vi "Group Channels By VS and MB Type.vi"(7 "Channel Type":T1, 8 "error in (no error)":errorcluster, 11 "Item Ref in":T2 format="%.0x") -> (0 "error out":errorcluster, 2 "Channels":T3, 3 "Device Ref out":T2 format="%.0x")   [LabVIEW 2019, in "Modbus Master System Explorer.lvlib"]
uses:
  Modbus Master System Explorer.lvlib
  Shared/Controls/Data Model/Channel Data.ctl
  Shared/Controls/Data Model/Channel.ctl
  SubVIs/Modbus Type.ctl
  <vilib>/NI VeriStand/Custom Device API/Custom Device Channel Type.ctl
  Shared/Controls/Data Model/Mapping.ctl
  Shared/Controls/Data Model/DataType.ctl
  <vilib>/NI VeriStand/Custom Device API/Custom Device Item Ref.ctl
  <vilib>/NI VeriStand/Custom Device API/Custom Device API.lvlib
  Shared/Modbus Master Shared.lvlib
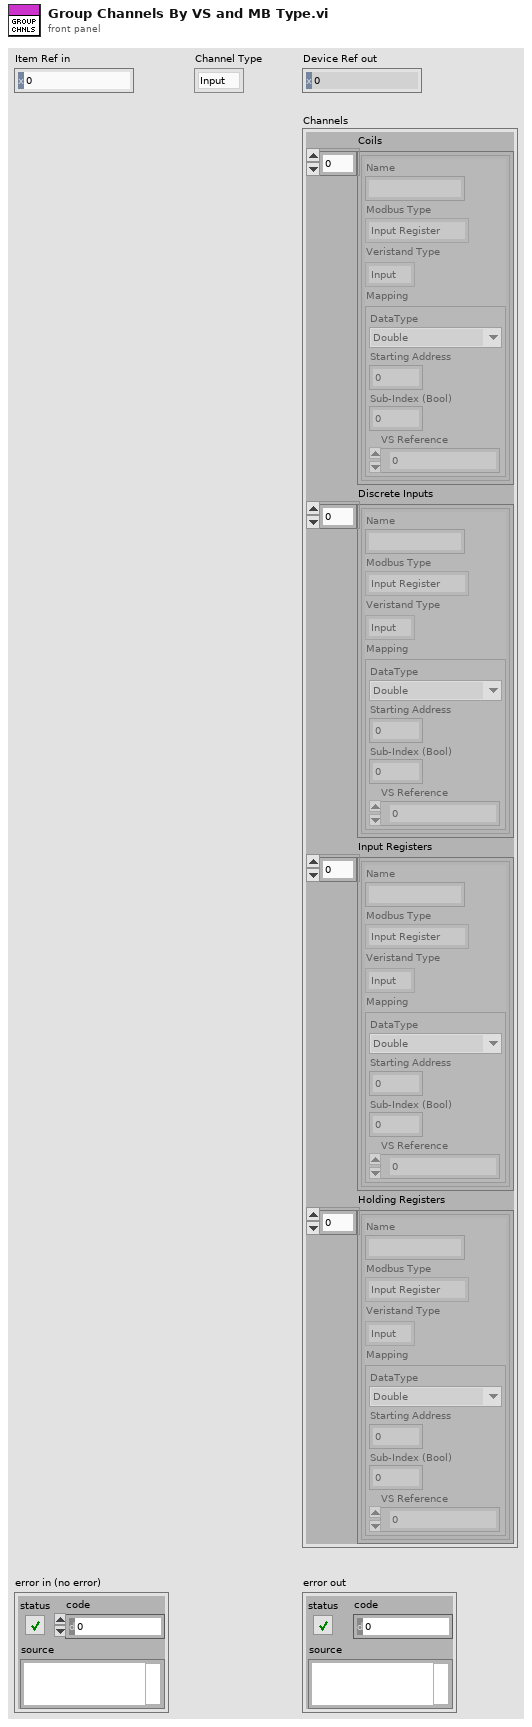
[diagram p1: front panel]
types:
  T1 = typedef "Custom Device API.lvlib/Custom Device Channel Type.ctl" = enum16{"Input", "Output"}
  T2 = typedef "Custom Device API.lvlib/Custom Device Item Ref.ctl" = u64
  T3 = typedef "Modbus Master Shared.lvlib/Channel Data.ctl" = cluster{"Coils":T4[], "Discrete Inputs":T4[], "Input Registers":T4[], "Holding Registers":T4[]}
  T4 = typedef "Modbus Master Shared.lvlib/Channel.ctl" = cluster{"Name":string, "Modbus Type":T5, "Veristand Type":T1, "Mapping":T6}
  T5 = typedef "Modbus Master Shared.lvlib/Modbus Type.ctl" = enum16{"Coil", "Discrete Input", "Holding Register", "Input Register"}
  T6 = typedef "Modbus Master Shared.lvlib/Mapping.ctl" = cluster{"DataType":T7, "Starting Address":u16, "Sub-Index (Bool)":u16, "VS Reference":T2}
  T7 = typedef "Modbus Master Shared.lvlib/DataType.ctl" = enum16{"Double", "Single", "I64", "I32", "I16", "I8", "U64", "U32", "U16", "U8", "Boolean"}
  T8 = typedef "Custom Device API.lvlib/Custom Device Item Info.ctl" = cluster{"Name":string, "Is Channel":bool, "GUID":string, "Is Waveform":bool}
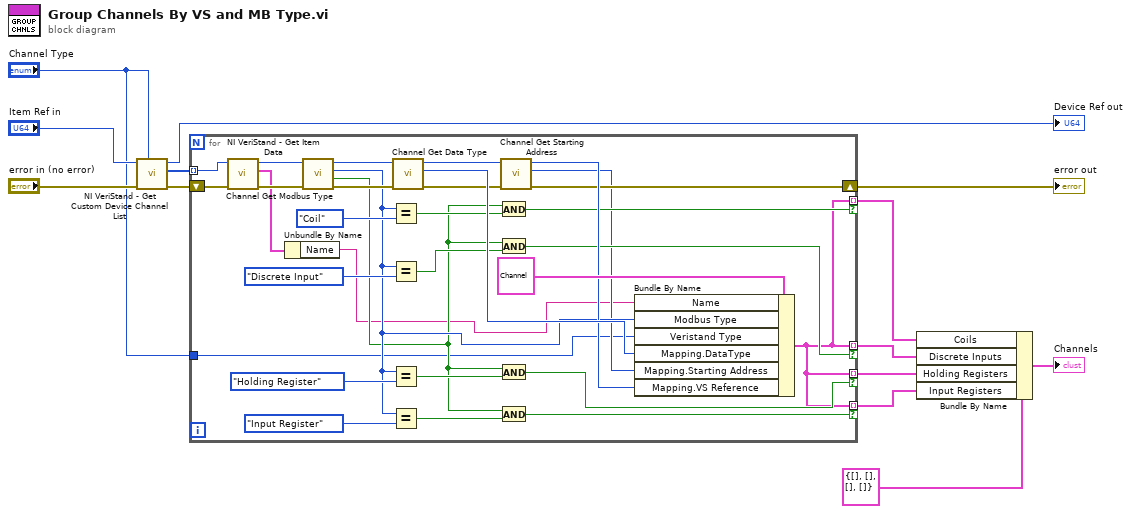
[diagram p0: block diagram]
diagram:
  n1 = call <vilib>:"NI VeriStand - Get Custom Device Channel List.vi"("Channel Type"="Channel Type", "error in (no error)"="error in (no error)", "Device Ref in"="Item Ref in") -> ("error out"=w3:errorcluster, "Specified Channel Ref List"=w1:T2[], "Device Ref out"=→"Device Ref out":T2)  [unwired: 6 in]
  n2 = for {
    tunnel: w1 -> [w15] mode=indexing
    tunnel: "Channel Type" -> [w16]
    tunnel: [w23] -> w10 mode=indexing if=w29
    tunnel: [w23] -> w11 mode=indexing if=w28
    tunnel: [w23] -> w12 mode=indexing if=w27
    tunnel: [w23] -> w13 mode=indexing if=w26
    shift-right: [w32] -> w8
    shift-left: w3 -> [w20]
    n3 = call <vilib>:"NI VeriStand - Get Item Data.vi"("error in (no error)"=w20, "Item Ref in"=w15) -> ("error out"=w19:errorcluster, "Item Info"=w18:T8, "Item Ref out"=w14:T2)  [unwired: 6 in, 1 out]
    n4 = Unbundle By Name(w18) -> ("Name"=w17:string)
    n5 = call "Channel Get Modbus Type.vi"("error in (no error)"=w19, "Channel Ref"=w14) -> ("error out"=w40:errorcluster, "Is MB Type?"=w25:bool, "Type"=w31:T5, "Item Ref out"=w43:T2)  [unwired: 6 in]
    n6 = Equal?(x=w31, y=Modbus_Type."Coil") -> (x = y?=w30:bool)
    n7 = Equal?(x=w31, y=Modbus_Type."Discrete Input") -> (x = y?=w35:bool)
    n8 = Equal?(x=w31, y=Modbus_Type."Holding Register") -> (x = y?=w34:bool)
    n9 = Equal?(x=w31, y=Modbus_Type."Input Register") -> (x = y?=w33:bool)
    n10 = call "Channel Get Data Type.vi"("error in (no error)"=w40, "Item Ref in"=w43) -> ("error out"=w22:errorcluster, "Data Type"=w42:T7, "Item Ref out"=w21:T2)  [unwired: 7 in]
    n11 = And(x=w25, y=w30) -> (x .and. y?=w29:bool)
    n12 = And(x=w25, y=w35) -> (x .and. y?=w28:bool)
    n13 = And(x=w25, y=w34) -> (x .and. y?=w27:bool)
    n14 = And(x=w25, y=w33) -> (x .and. y?=w26:bool)
    n15 = call "Channel Get Starting Address.vi"("error in (no error)"=w22, "Item Ref in"=w21) -> ("error out"=w32:errorcluster, "Value"=w24:u16, "Item Ref out"=w41:T2)  [unwired: 7 in]
    n16 = Bundle By Name(cluster=T4 {"Name"="", "Modbus Type"=enum."Input Register", "Veristand Type"=enum."Input", "Mapping"={"DataType"=enum."Boolean", "Starting Address"=0, "Sub-Index (Bool)"=0, "VS Reference"=0}} ("Channel"), "Name"=w17, "Modbus Type"=w31, "Veristand Type"=w16, "Mapping.DataType"=w42, "Mapping.Starting Address"=w24, "Mapping.VS Reference"=w41) -> (w23:T4)
  }
  "error out" <- w8
  n17 = Bundle By Name(cluster=T3 {"Coils"=[], "Discrete Inputs"=[], "Input Registers"=[], "Holding Registers"=[]} ("Outputs"), "Coils"=w10, "Discrete Inputs"=w11, "Holding Registers"=w12, "Input Registers"=w13) -> (→"Channels":T3)
